vi "PicoScopeospaGetValues.vi"(7 "Buffer and Transfer Settings":T1={"startIndex"=0, "Samples"=1000, "Down Sample Ratio"=1, "Down-Sample Mode"=1} {"Down-Sample Mode" items=["RAW none"=2147483648, "None"=0, "Aggregate"=1, "Decimate"=2, "Average"=4]; "Down Sample Ratio" step=1; "Samples" format="%_6p"}, 8 "error in (no error)":errorcluster, 11 "handle in":i16) -> (0 "error out":errorcluster, 3 "handle out":i16, 4 "overflow":i16 format="%010b", 6 "noOfSamples":u64)   [LabVIEW 2010]
doc: "Calls GetValues"
uses:
  psospa.dll
  shared/Buffer and Transfer Settings.ctl
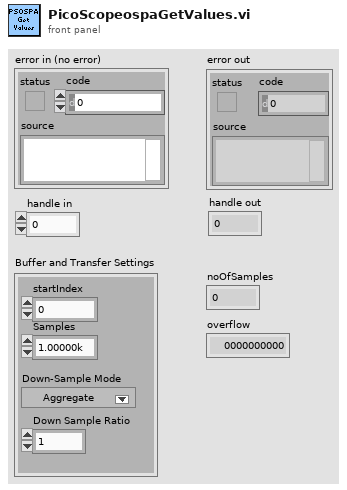
[diagram p1: front panel]
types:
  T1 = typedef "Buffer and Transfer Settings.ctl" = cluster{"startIndex":u64, "Samples":u64, "Down Sample Ratio":u64, "Down-Sample Mode":u32}
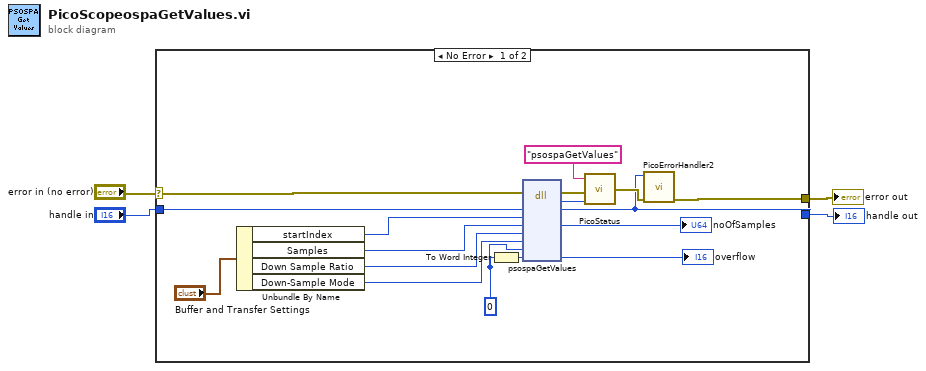
[diagram p0: block diagram]
diagram:
  n1 = case shown="No Error" "error in (no error)" {
    selector: "error in (no error)" -> [w9 w22]
    tunnel: "handle in" -> [w8 w23]
    tunnel: [w6 w23] -> w4
    tunnel: [w7 w22] -> w3
    frame No Error {
      w13 = u64 0 ("overflow")
      n2 = Unbundle By Name("Buffer and Transfer Settings") -> ("startIndex"=w10:u64, "Samples"=w21:u64, "Down Sample Ratio"=w17:u64, "Down-Sample Mode"=w18:u32)
      n3 = To Word Integer(number=w13) -> (16bit integer=w19:i16)
      n4 = dll-call lib="psospa.dll" fn="psospaGetValues" ("ps3000.dll:_ps3000_open_unit@0")(error in=w9, "handle"=w8, "startIndex"=w10, "noOfSamples"=w21, "downSampleRatio"=w17, "downSampleRatioMode"=w18, "segmentIndex"=w13, "overflow"=w19) -> (error out=w16:errorcluster, "PICO_STATUS"=w15:u32, "handle"=w6:i16, "noOfSamples"=→"noOfSamples":u64, "overflow"=→"overflow":i16)  [unwired: 6 in, 1 out]
      n5 = call "PicoStatus.vi"("PICO STATUS"=w15, "error in"=w16, "source"="psospaGetValues") -> ("error out"=w20:errorcluster)
      n6 = call "PicoErrorHandler2.vi"("error in (no error)"=w20, "handle In"=w6) -> ("error out"=w7:errorcluster)  [unwired: 9 in]
    }
    frame Error {
    }
  }
  "error out" <- w3
  "handle out" <- w4
